vi "ArduinoAutoDetect.vi"(8 "error in (no error)":errorcluster, 11 "Visa Resource":refnum<visa-resource-name>) -> (0 "error out":errorcluster, 3 "VISA resource":refnum<visa-resource-name>)   [LabVIEW 2019, in "ArduinoControl.lvclass"]
uses:
  ArduinoControl.lvclass
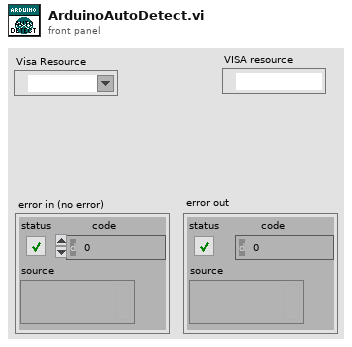
[diagram p1: front panel]
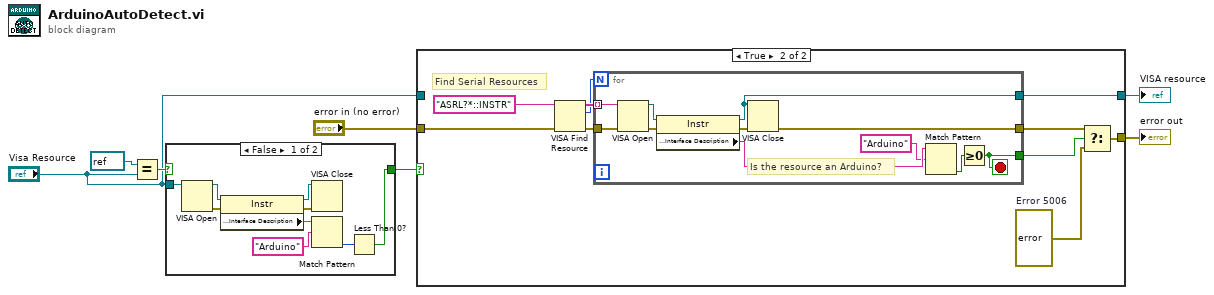
[diagram p0: block diagram]
diagram:
  n1 = Equal?(x=refnum<visa-resource-name> refnum ("VISA resource"), y="Visa Resource") -> (x = y?=w3:bool)
  n2 = case shown="False" w3 {
    selector: w3 -> [_ w17]
    tunnel: [w8 w17] -> w1
    tunnel: "Visa Resource" -> [w10 _]
    frame False {
      n3 = VISA Open(VISA resource name=w10) -> (VISA resource name=w11:refnum<visa-resource-name>, error out=w13:errorcluster)  [unwired: 4 in]
      n4 = property class="Instr"(reference=w11, error in=w13) -> (reference out=w16:refnum<visa-resource-name>, error out=w12:errorcluster, "Interface Information:Interface Description"=w15:string)
      n5 = VISA Close(VISA resource name=w16, error in (no error)=w12) -> ()  [unwired: 1 out]
      n6 = Match Pattern(string=w15, regular expression="Arduino") -> (offset past match=w9:i32)  [unwired: 1 in, 3 out]
      n7 = Less Than 0?(x=w9) -> (x < 0?=w8:bool)
    }
    frame True {
    }
  }
  n8 = case shown="True" w1 {
    tunnel: "error in (no error)" -> [w18 w22]
    tunnel: [w18 w21] -> w6
    tunnel: [w19 w20] -> w5
    tunnel: "Visa Resource" -> [w19 _]
    frame False {
    }
    frame True {
      w29 = errorcluster {"status"=TRUE, "code"=5005, "source"="Unable to find Arduino.  Please make sure the Arduino is connected to your system and that the Arduino drivers are installed."}  # Error 5006
      # "Find Serial Resources"
      n9 = VISA Find Resource(8:w22, 11:"ASRL?*::INSTR" ("expression (\"\")")) -> (0:w26:errorcluster, 2:w24:u32, 3:w25:string[])  [unwired: 1 in]
      n10 = for {
        N: w24 -> [_]
        tunnel: w25 -> [w30] mode=indexing
        tunnel: w26 -> [w34]
        tunnel: [w33] -> w28
        tunnel: [w32] -> w20
        tunnel: [w31] -> w27
        stop <- w31 stop-if-true
        # "Is the resource an Arduino?"
        n11 = VISA Open(error in (no error)=w34, VISA resource name=w30) -> (VISA resource name=w35:refnum<visa-resource-name>, error out=w40:errorcluster)  [unwired: 3 in]
        n12 = property class="Instr"(reference=w35, error in=w40) -> (reference out=w32:refnum<visa-resource-name>, error out=w39:errorcluster, "Interface Information:Interface Description"=w38:string)
        n13 = VISA Close(VISA resource name=w32, error in (no error)=w39) -> (error out=w33:errorcluster)
        n14 = Match Pattern(string=w38, regular expression="Arduino") -> (offset past match=w36:i32)  [unwired: 1 in, 3 out]
        n15 = Greater Or Equal To 0?(x=w36) -> (x >= 0?=w31:bool)
      }
      n16 = Select(t=w28, s=w27, f=w29) -> (s? t:f=w21:errorcluster)
    }
  }
  "error out" <- w6
  "VISA resource" <- w5
